vi "Configure List Recorder.vi"(8 "error in":errorcluster, 9 "Parameter":T1={"Wave Type"=0, "Level(%)"=1.0, "Vac(V)"=0.0, "Vdc(V)"=0.0, "Freq(Hz)"=0.0, "Time(ms)"=0, "Start Phase(°)"=0.0, "Stop Phase(°)"=0.0, "Kac"=0.0, "Kdc"=0.0, "Kfreq"=0.0, "Repeat"=1} {"Repeat" min=1 max=50000 step=1; "Kfreq" min=0.0; "Kdc" min=0.0; "Kac" min=0.0; "Stop Phase(°)" min=0.0 max=360.0; "Start Phase(°)" min=0.0 max=360.0; "Time(ms)" max=100000000; "Freq(Hz)" min=0.0; "Vdc(V)" min=0.0; "Vac(V)" min=0.0; "Level(%)" min=0.0 max=100.0; "Wave Type" max=39 step=1}, 10 "Step":u32=1 min=1 max=50 step=1, 11 "VISA resource name":refnum<visa-resource-name>) -> (0 "error out":errorcluster, 3 "VISA resource name out":refnum<visa-resource-name>)   [LabVIEW 2015, in "IT-M7700.lvlib"]
doc: "This command is used to set the logging parameters of a single Step in a List. Record parameter format for: Step index value, \"Type, Wave Type, Level, Vac, Vdc, Freq, Time, Start Phase, StopPhase, Kac, Kdc, Kfreq, Repeat.\" The delay for running this command is 50ms.\n<b>Step</b>\n1-50\n<b>Wave Type</b>\n0-39\n 0: Sine\n 1: Square\n 2: Triangle\n 3: Saw\n 4: Clip Sine\n 5~34: THD1~THD30\n 35~39: USER1~USER5\n<b>Level(%)</b>\n0-100\n<b>Vac(V)</b>\n0-MAX\n<b>Vdc(V)</b>\n0-MAX\n<b>Freq(Hz)</b>\n0-MAX\n<b>Time(ms)</b>\n0-100000000\n<b>Start Phase(°)</b>\n0-360\n<b>Stop Phase(°)</b>\n0-360\n<b>Kac</b>\n0-MAX\n<b>Kdc</b>\n0-MAX\n<b>Kfreq</b>\n0-MAX\n<b>Repeat</b>\n1-50000"
uses:
  <instrlib>/IT-M7700/IT-M7700.lvlib
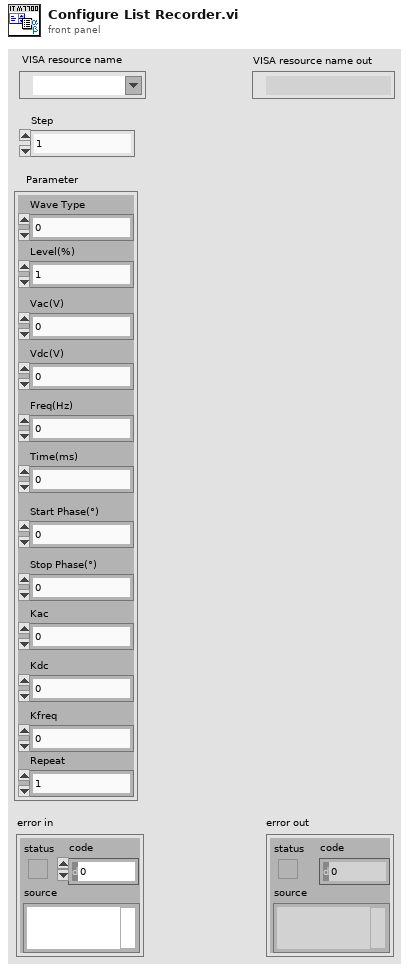
[diagram p1: front panel]
types:
  T1 = cluster{"Wave Type":u32, "Level(%)":dbl, "Vac(V)":dbl, "Vdc(V)":dbl, "Freq(Hz)":dbl, "Time(ms)":u32, "Start Phase(°)":dbl, "Stop Phase(°)":dbl, "Kac":dbl, "Kdc":dbl, "Kfreq":dbl, "Repeat":u32}
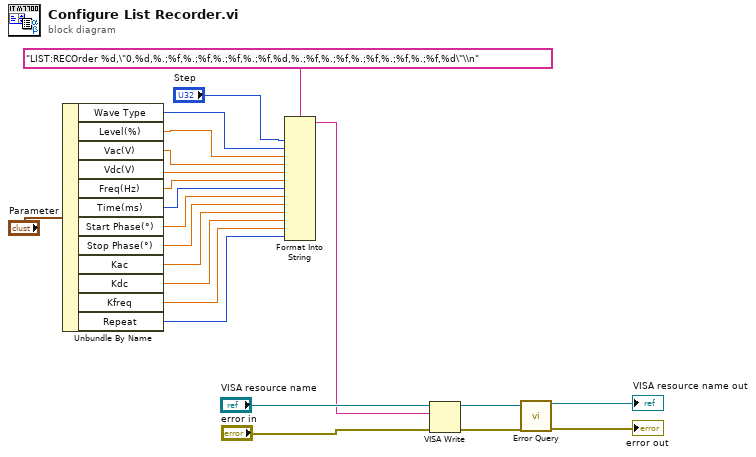
[diagram p0: block diagram]
diagram:
  n1 = Unbundle By Name("Parameter") -> ("Wave Type"=w17:u32, "Level(%)"=w16:dbl, "Vac(V)"=w15:dbl, "Vdc(V)"=w14:dbl, "Freq(Hz)"=w13:dbl, "Time(ms)"=w12:u32, "Start Phase(°)"=w11:dbl, "Stop Phase(°)"=w10:dbl, "Kac"=w9:dbl, "Kdc"=w8:dbl, "Kfreq"=w7:dbl, "Repeat"=w6:u32)
  n2 = Format Into String(format string="LIST:RECOrder %d,\"0,%d,%.;%f,%.;%f,%.;%f,%.;%f,%d,%.;%f,%.;%f,%.;%f,%.;%f,%.;%f,%d\"\\n", "Step", w17, w16, w15, w14, w13, w12, w11, w10, w9, w8, w7, w6) -> (resulting string=w19:string)  [unwired: 2 in, 1 out]
  n3 = VISA Write(VISA resource name="VISA resource name", write buffer=w19, error in (no error)="error in") -> (VISA resource name out=w5:refnum<visa-resource-name>, error out=w4:errorcluster)  [unwired: 1 out]
  n4 = call <instrlib>:"Error Query.vi"("error in"=w4, "VISA resource name"=w5) -> ("error out"=→"error out":errorcluster, "VISA resource name out"=→"VISA resource name out":refnum<visa-resource-name>)  [unwired: 6 in, 2 out]
